vi "Format Response for Log.vi"(3 "error in":errorcluster, 4 "Response":string, 5 "Command":T1) -> (0 "error out":errorcluster, 1 "Stim RSP for Log":string, 2 "Command":T1)   [LabVIEW 2019]
uses:
  Bits Library/Get Bits (U8).vi
  Bits Library/Get Bit (U8).vi
  Bits Library/Bits.lvlib
panel:
  out "String":string
  out "Rsp string byte array":u8[](array[numeric]) format="%08b"
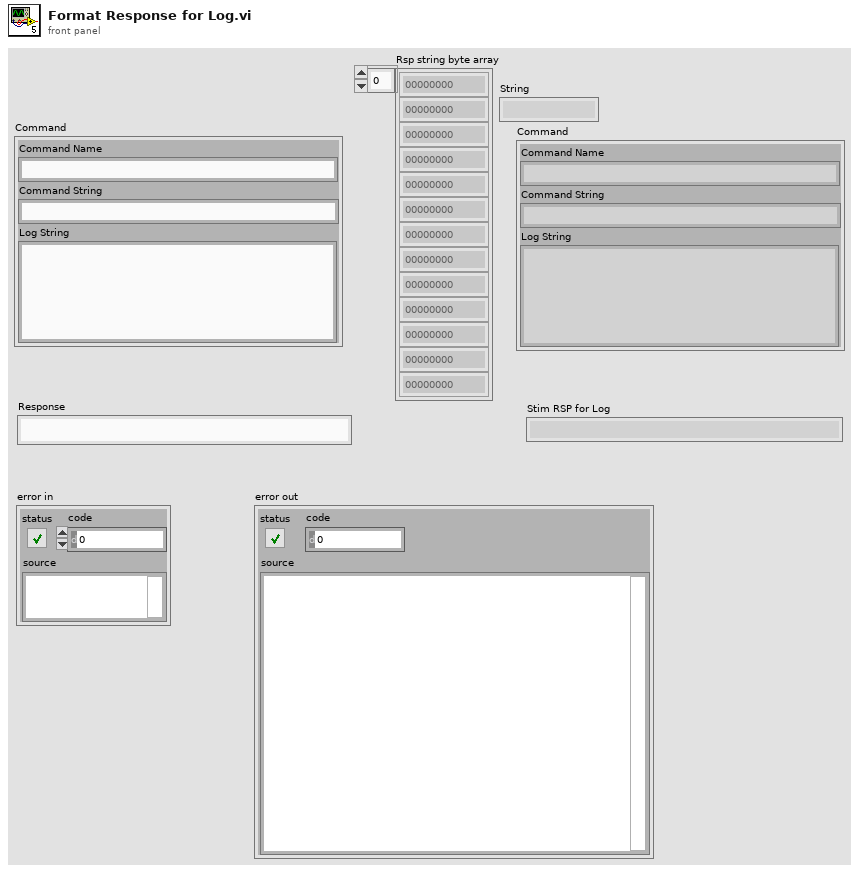
[diagram p1: front panel]
types:
  T1 = cluster{"Command Name":string, "Command String":string, "Log String":string}
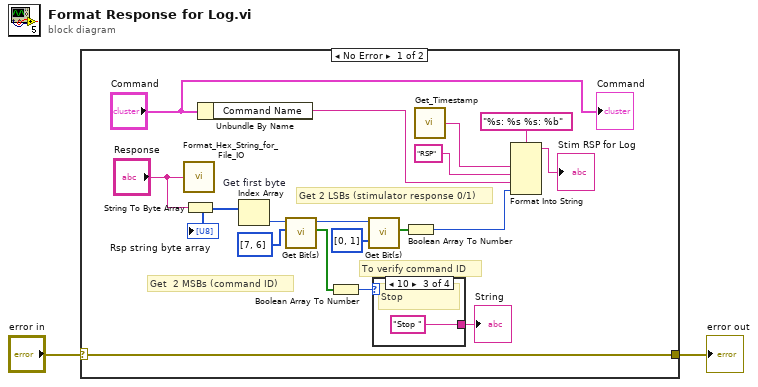
[diagram p0: block diagram]
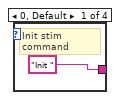
[diagram p2: hidden frame]
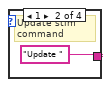
[diagram p3: hidden frame]
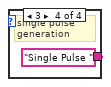
[diagram p4: hidden frame]
diagram:
  n1 = case shown="No Error" "error in" {
    selector: "error in" -> [w19 w25]
    tunnel: [w19 w25] -> w1
    frame No Error {
      # "Get 2 LSBs (stimulator response 0/1)"
      # "To verify command ID"
      # "Get  2 MSBs (command ID)"
      n2 = call "Format_Hex_String_for_File_IO.vi"("Hex String in"="Response") -> ()  [unwired: 1 out]
      n3 = String To Byte Array(string="Response") -> (unsigned byte array=w18:u8[])
      "Rsp string byte array" <- w18
      n4 = Unbundle By Name("Command") -> ("Command Name"=w6:string)
      n5 = Index Array "Get first byte"(array=w18) -> (element=w13:u8)  [unwired: 1 in]
      n6 = call-poly "Get Bit(s).vi"("Bits"=u8[] [7, 6], "Number"=w13) -> ("Values"=w12:bool[], "Number Out"=w10:u8)  [unwired: 8 in]
      n7 = Boolean Array To Number(Boolean array=w12) -> (number=w11:u32)
      n8 = call-poly "Get Bit(s).vi"("Bits"=u8[] [0, 1], "Number"=w10) -> ("Values"=w15:bool[])  [unwired: 8 in, 1 out]
      n9 = case shown="10" w11 {
        tunnel: ["Init " "Update " "Stop " "Single Pulse "] -> w9
        frame 0, Default {
          # "Init stim command"
        }
        frame 1 {
          # "Update stim command"
        }
        frame 2 {
          # "Stop"
        }
        frame 3 {
          # "single pulse generation"
        }
      }
      "String" <- w9
      n10 = Boolean Array To Number(Boolean array=w15) -> (number=w5:u32)
      n11 = call "Get_Timestamp.vi"() -> ("date/time string"=w8:string)  [unwired: 1 in]
      n12 = Format Into String(format string="%s: %s %s: %b", w8, "RSP" ("Tag"), w6, w5) -> (resulting string=→"Stim RSP for Log":string)  [unwired: 2 in, 1 out]
      "Command" <- "Command"
    }
    frame Error {
    }
  }
  "error out" <- w1
